vi "pcap flush.vi"(8 "error in":errorcluster, 11 "pcap_dumper_t in":u64) -> (0 "error out":errorcluster, 3 "pcap_dumper_t out":u64)   [LabVIEW 2020, in "libpcaplv.lvlib"]
uses:
  libpcaplv.lvlib
  <vilib>/Utility/sysdir.llb/Get System Directory.vi
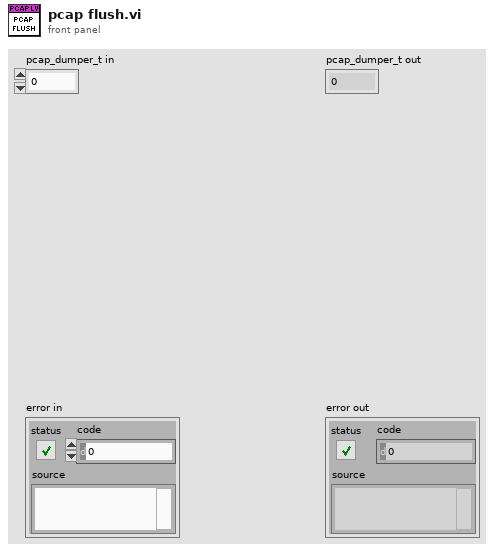
[diagram p1: front panel]
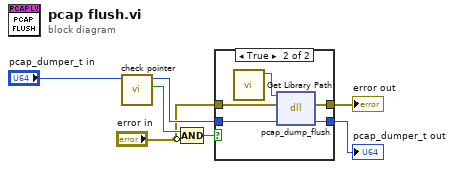
[diagram p0: block diagram]
diagram:
  n1 = call "check pointer.vi"("pointer in"="pcap_dumper_t in") -> ("ok"=w6:bool, "pointer out"=w4:u64)  [unwired: 9 in]
  n2 = Compound Arithmetic op=AND(w6, invert "error in") -> (w3:bool)
  n3 = case shown="True" w3 {
    tunnel: [w8 w11] -> w7
    tunnel: w4 -> [w9 w13]
    tunnel: "error in" -> [w8 w14]
    tunnel: [w9 w12] -> w1
    frame False {
    }
    frame True {
      n4 = call "Get Library Path.vi"() -> ("library path"=w10:path)  [unwired: 11 in]
      n5 = dll-call lib="libpcap.*" fn="pcap_dump_flush"(path in=w10, error in=w14, "pcap_dumper_t"=w13) -> (error out=w11:errorcluster, "pcap_dumper_t"=w12:u64)  [unwired: 2 in, 1 out]
    }
  }
  "pcap_dumper_t out" <- w1
  "error out" <- w7
